vi "solar_misc Rendezvous Destroy.vi"(8 "error in (no error)":errorcluster, 9 "Force Destroy? (F)":bool, 11 "Rendezvous in":refnum<queue>) -> (0 "error out":errorcluster)   [LabVIEW 2018]
doc: "This is a simplified version of NI's rendezvous destroy VI."
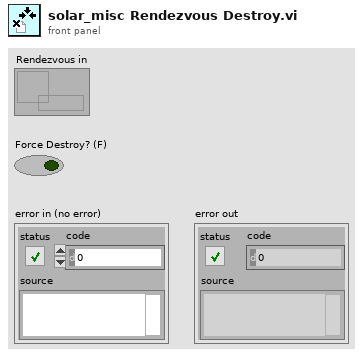
[diagram p1: front panel]
types:
  T1 = cluster{"Size":u32, "Rendezvous":refnum<queue>[]}[]
  T2 = cluster{"Size":u32, "Rendezvous":refnum<queue>[]}
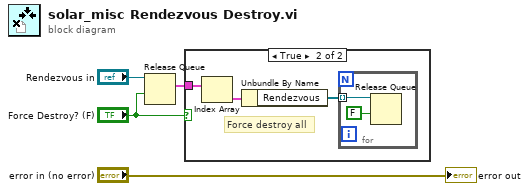
[diagram p0: block diagram]
diagram:
  n1 = Release Queue(queue="Rendezvous in", force destroy? (F)="Force Destroy? (F)") -> (remaining elements=w2:T1)  [unwired: 1 in, 2 out]
  n2 = case shown="True" "Force Destroy? (F)" {
    tunnel: w2 -> [_ w7]
    frame False {
    }
    frame True {
      # "Force destroy all"
      n3 = Index Array(array=w7) -> (element=w6:T2)  [unwired: 1 in]
      n4 = Unbundle By Name(w6) -> ("Rendezvous"=w5:refnum<queue>[])
      n5 = for {
        tunnel: w5 -> [w9] mode=indexing
        n6 = Release Queue(queue=w9, force destroy? (F)=FALSE) -> ()  [unwired: 1 in, 3 out]
      }
    }
  }
  "error out" <- "error in (no error)"
